vi "Read yellow_cards.vi"(8 "error in (no error)":errorcluster, 11 "Team in":refnum<class "Team.lvclass">) -> (0 "error out":errorcluster, 2 "yellow_cards":i32, 3 "Team out":refnum<class "Team.lvclass">)   [LabVIEW 2023, in "Team.lvclass"]
uses:
  Team.lvclass
  Team.lvclass/Team.ctl
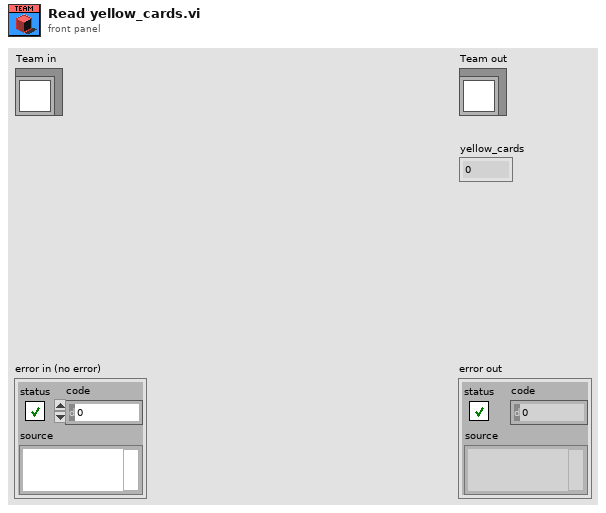
[diagram p1: front panel]
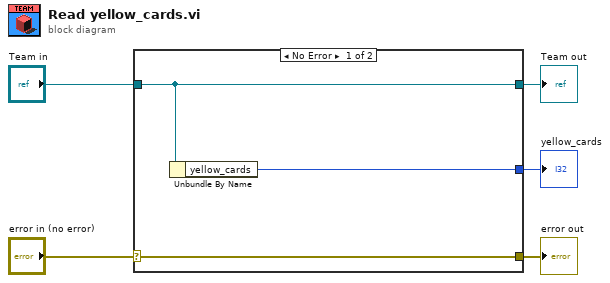
[diagram p0: block diagram]
diagram:
  n1 = case shown="No Error" "error in (no error)" {
    selector: "error in (no error)" -> [w8 w9]
    tunnel: [w8 w9] -> w4
    tunnel: [w7 w10] -> w2
    tunnel: "Team in" -> [w7 w10]
    tunnel: [w6 _] -> w1
    frame No Error {
      n2 = Unbundle By Name(w7) -> ("yellow_cards"=w6:i32)
    }
    frame Error {
    }
  }
  "error out" <- w4
  "Team out" <- w2
  "yellow_cards" <- w1
